vi "synnax writer close.vi"(8 "error in":errorcluster, 11 "writer":u64) -> (0 "error out":errorcluster)   [LabVIEW 2026, in "synnax_clib.lvlib"]
doc: "SYNNAX_EXPORT int32_t synnax_writer_close(SynnaxWriter writer, SynnaxError err);"
uses:
  synnax_clib.lvlib
  synnax_clib.dll
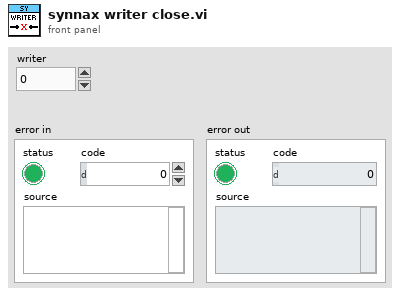
[diagram p1: front panel]
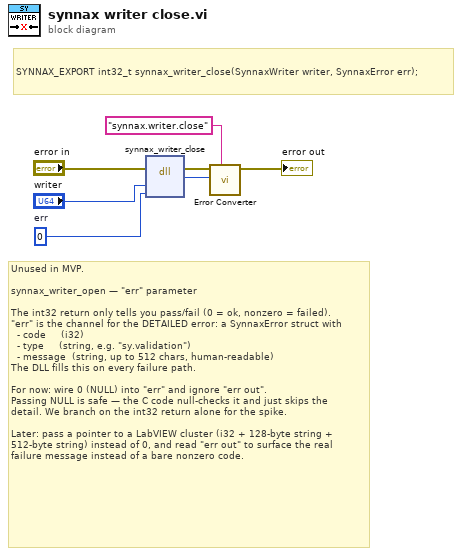
[diagram p0: block diagram]
diagram:
  w6 = u64 0  # err
  # "Unused in MVP.\n\nsynnax_writer_open — \"err\" parameter\n\nThe int32 return only tells you pass/fail (0 = ok, nonzero = failed).\n\"err\" is the channel for the DETAILED error: a SynnaxError struct with\n  - code     (i32)\n  - type     (string, e.g. \"sy.validation\")\n  - message  (string, up to 512 chars, human-readable)\nThe DLL fills this on every failure path.\n\nFor now: wire 0 (NULL) into \"err\" and ignore \"err out\".\nPassing NULL is safe — the C code null-checks it and just skips the\ndetail. We branch on the int32 return alone for the spike.\n\nLater: pass a pointer to a LabVIEW cluster (i32 + 128-byte string +\n512-byte string) instead of 0, and read \"err out\" to surface the real\nfailure message instead of a bare nonzero code."
  # "SYNNAX_EXPORT int32_t synnax_writer_close(SynnaxWriter writer, SynnaxError err);"
  n1 = dll-call lib="C/synnax/client/labview/synnax_clib.*" fn="synnax_writer_close"(error in="error in", "writer"="writer", "err"=w6) -> (error out=w5:errorcluster, w4:i32)  [unwired: 4 in, 1 out]
  n2 = call "Error Converter.vi"("source"="synnax.writer.close", "error code"=w4, "error in (no error)"=w5) -> ("error out"=→"error out":errorcluster)  [unwired: 8 in]
